vi "st_voltmetr.vi"() -> ()   [LabVIEW 2017]
uses:
  <vilib>/Analysis/4window.llb/windowTd.ctl
  controls/A5000_param.ctl
  subVIs/st_str Global.vi
  <vilib>/measure/maspectr.llb/FFT Spectrum (Mag-Phase) for N Chan.vi
  <vilib>/Utility/file.llb/Read Delimited Spreadsheet (string).vi
  <vilib>/measure/NI_MAPro.lvlib
  <vilib>/Analysis/NI_AALPro.lvlib
panel:
  out "Waveform Spectrogramm":cluster{"f0":dbl, "df":dbl, "magnitude":dbl[]}[](graph)
  in  "window":T1=1 items=["Rectangle"=0, "Hanning"=1, "Hamming"=2, "Blackman-Harris"=3, "Exact Blackman"=4, "Blackman"=5, "Flat Top"=6, "4 Term B-Harris "=7, "7 Term B-Harris"=8, "Low Sidelobe"=9, "Blackman Nuttall"=11, "Triangle"=30, "Bartlett-Hanning"=31, "Bohman"=32, "Parzen"=33, "Welch"=34, "Kaiser"=60, "Dolph-Chebyshev"=61, "Gaussian"=62]
  out "comm?":bool
  out "ItemTag":string
  out "substring before match":string
  out "ItemPath":string
  in  "VChGEN":dbl=0.03 caption="Uскз канал \"GEN\", В" min=0.02 max=1.0 step=0.01 format="%.2f"
  in  "FGen":dbl=10.0 caption="Частота, кГц" min=0.01 max=500.0 step=0.01 format="%_4g"
  in  "GenEnb":bool
  in  "AutoFindFreqChB":bool
  in  "AutoFindFreqChA":bool
  in  "FChB":dbl=10.0 caption="Частота \"B\", кГц" format="%_4g"
  in  "FChA":dbl=10.0 caption="Частота \"A\", кГц" min=0.01 max=500.0 step=0.01 format="%_4g"
  out "VChB":dbl caption="Uскз канал \"B\", В" format="%.3f"
  out "VChA":dbl caption="Uскз канал \"A\", В" format="%.3f"
  in  "RangeChB":T2(ring)=enum."10 В" caption="Диапазон \"B\""
  in  "RangeChA":T3(ring)=enum."10 В" caption="Диапазон \"A\""
  in  "View":T4(ring)
  in  "Protocol":string[][](table)=[["11.02.26 11:54:00", "3.0012e-3", "3.0012e-3", "125,65", "125,65", "1 В", "1 В"], ["", "", "", "", "", "", ""]]
  in  "Checkbox":bool
  out "Waveform Oscillogram":waveform(dbl)[](graph)
  in  "Stop":bool
  in  "Capture":bool=TRUE
  out "overflow":i16
  out "noOfSamples":u32
  in  "Capture":bool
  in  "Tab Control":enum32{"Page 1"}(tab)
  out "OscCon":bool
  in  "Save":bool
  in  "Remove":bool
  in  "Add":bool
  in  "Report":bool
  in  "Delete":bool
  in  "Start Tool":bool
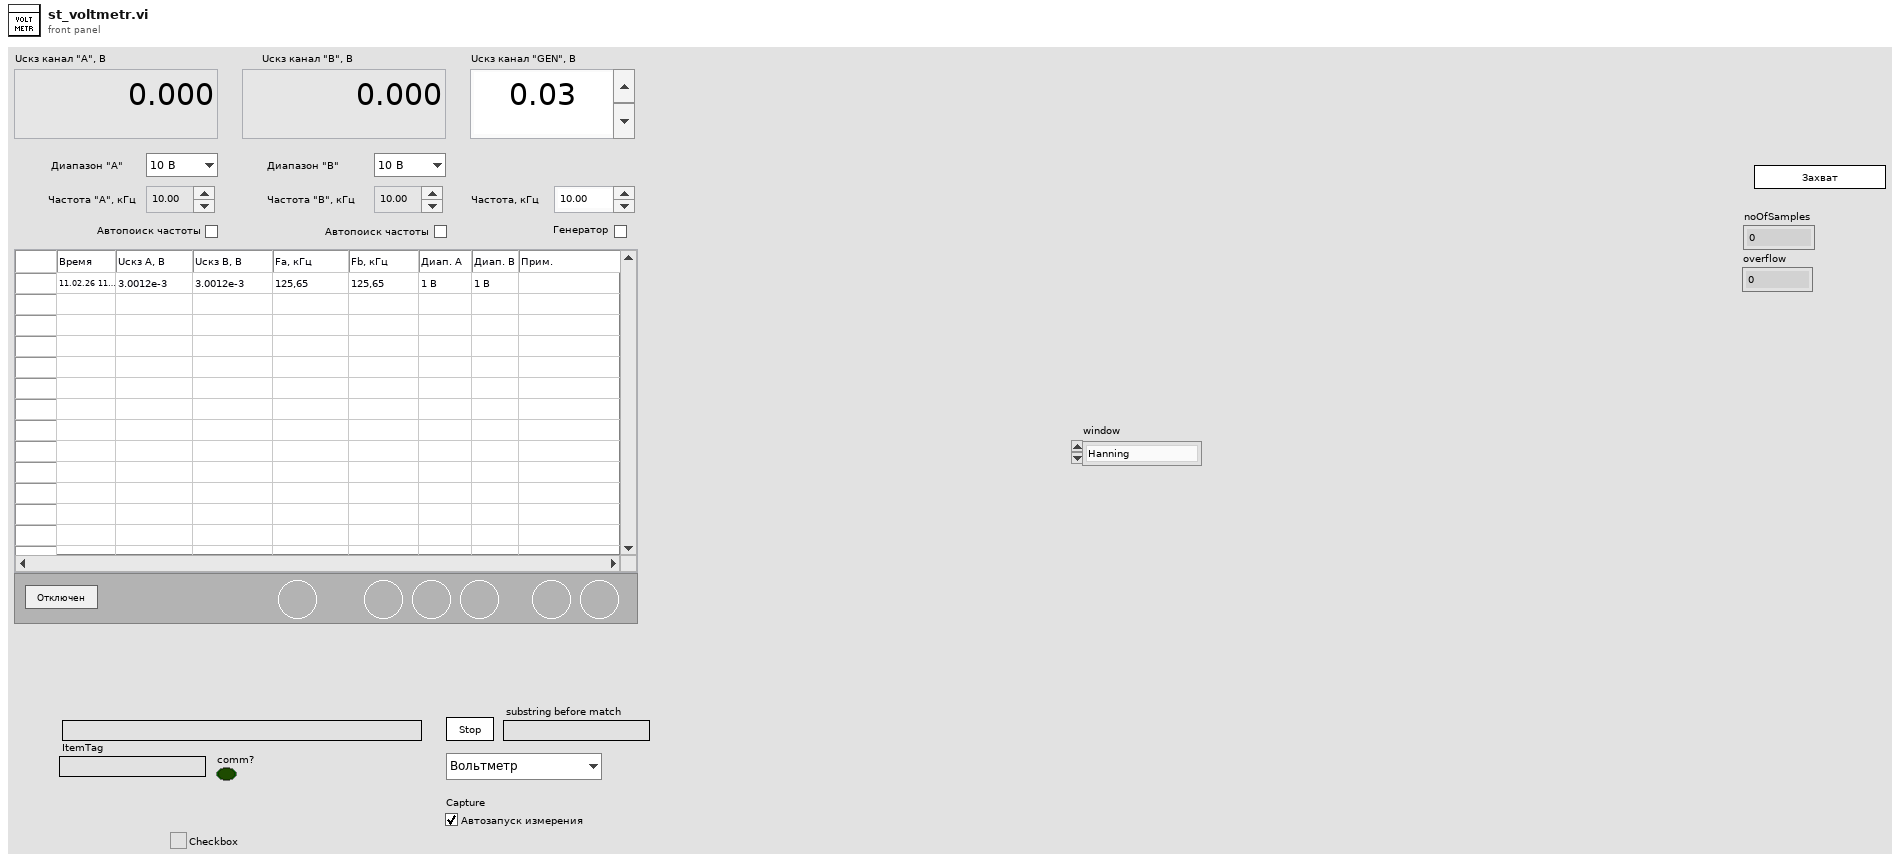
[diagram p1: front panel]
types:
  T1 = typedef "NI_AALPro.lvlib/windowTd.ctl" = u32
  T2 = enum16{"5 мВ", "10 мВ", "25 мВ", "50 мВ", "100 мВ", "250 мВ", "0,5 В", "1 В", "2,5 В", "5 В", "10 В", "Авто", "Выкл."}
  T3 = enum16{"5 мВ", "10 мВ", "25 мВ", "50 мВ", "100 мВ", "250 мВ", "0,5 В", "1,0 В", "2,5 В", "5 В", "10 В", "Авто", "Выкл."}
  T4 = enum16{"Вольтметр", "Осциллограмма", "Спектрограмма"}
  T5 = typedef "A5000_param.ctl" = cluster{"ChannelA":cluster{"Enabled":bool, "Coupling":i16, "Range":u16, "Analogue Offset":sgl}, "ChannelB":cluster{"Enabled":bool, "Coupling":i16, "Range":u16, "Analogue Offset":sgl}, "Trigger":cluster{"Trigger Enabled":bool, "Trigger Source":enum16{"Channel A", "Channel B", "Channel C", "Channel D", "Ext."}, "Trigger Threshold (volts)":dbl, "Trigger Direction":u16, "Trigger Delay (samples)":u32, "Auto Trigger Time (ms)":i16}, "MaxADCvalue":i16, "handle":i16, "Acquisition":cluster{"preTriggerSamples":i32, "postTriggerSamples":i32, "timebase":u32, "Down-Sample Mode":u32, "Down Sample Ratio":u32}, "Device Info":cluster{"Driver Version":string, "USB Version":string, "Hardware":string, "Variant":string, "Batch and Serial":string, "Cal Date":string, "Kernel Version":string, "Digital HW Version":string, "Analogue HW Version":string, "MSO":bool, "Number of channels":i16}, "Properties":cluster{"Sample Frequency":sgl, "Sample Rate":sgl, "Max Samples Available":i32, "Number of Samples":u32, "Total Capture Time (sec) ":sgl, "Max Total Capture Time Available (sec)":sgl}, "Resolution":i32, "EmulateV":bool, "General AWG Settings":cluster{"Peak-to-Peak Voltage (microvolts)":u32, "Offset Voltage (microvolts)":i32, "Wave Type":u32, "Sweep Type":u32, "Shots":u32, "Sweeps":u32, "Trigger Type":u32, "Trigger Source":u32, "Ext. Threshold (ADC count)":i16, "White Noise/PRBS":u32}, "Standard Waveform Settings":cluster{"Start Frequency":dbl, "Stop Frequency":dbl, "Increment":dbl, "Dwell Time (seconds)":dbl}, "Arbitrary Waveform Settings":cluster{"Arbirary waveform file path":path, "Index Mode":u32}, "AutoDiapChA":bool, "AutoDiapChB":bool}
  T6 = cluster{"AutoFindFreqChA":bool, "AutoFindFreqChB":bool, "FChA":dbl, "FChB":dbl}
  T7 = cluster{"dB On (F)":bool, "unwrap phase (F)":bool, "convert to degree (F)":bool}
  T8 = enum8{"Enabled", "Disabled", "Disabled and Grayed Out"}
  T9 = cluster{"Версия:":string, "Наименование ПО:":string, "Год выпуска:":string, "Производитель:":string, "MD5":string, "Наименование ПО полное:":string, "Build":string}
  T10 = typedef "LVRowAndColumnTypeDef.ctl" = cluster{"Row":i32, "Column":i32}
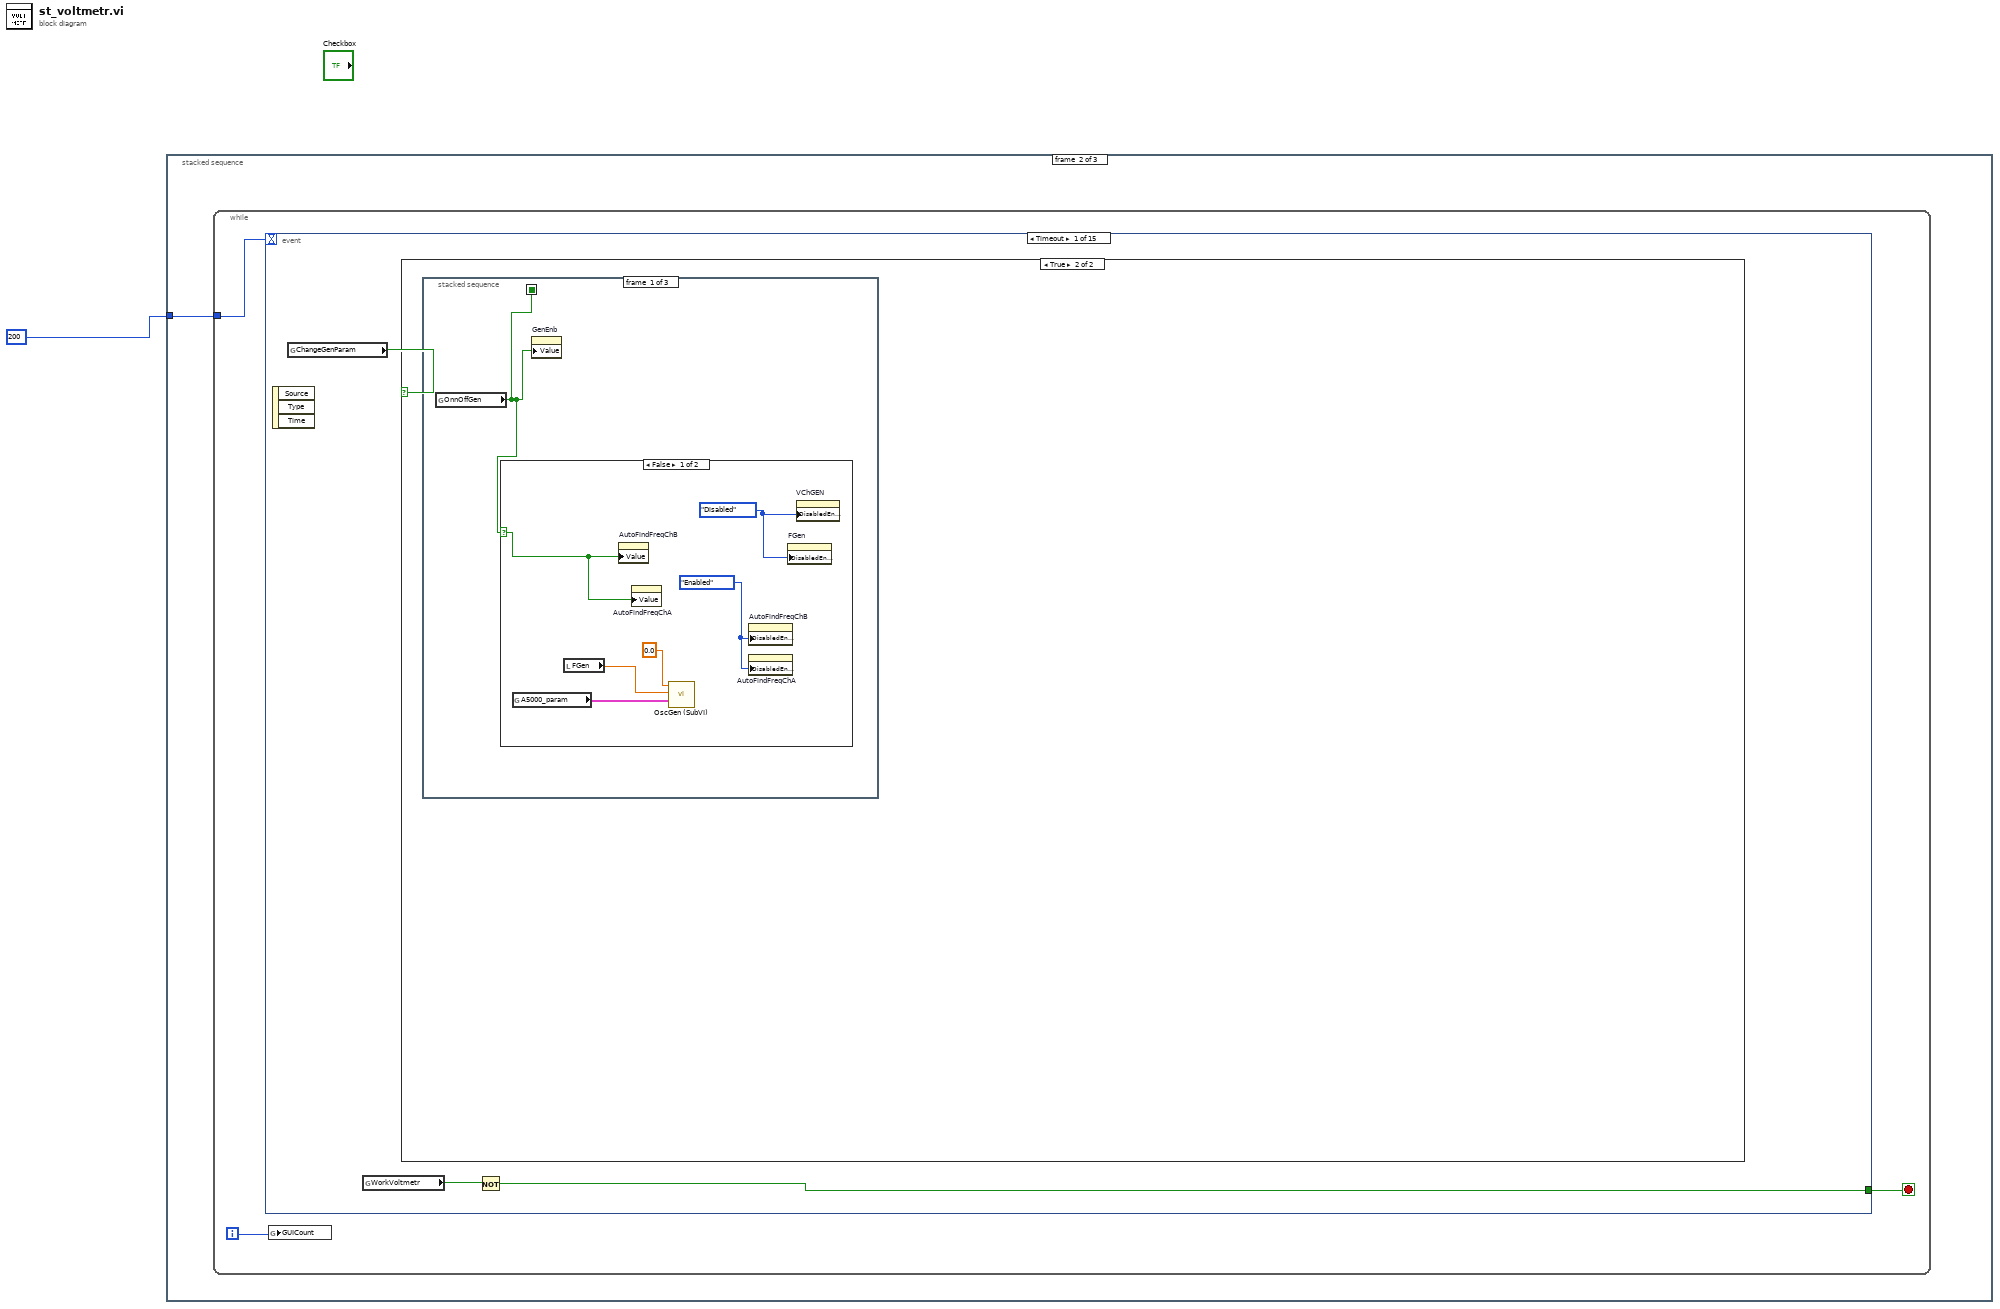
[diagram p0: block diagram]
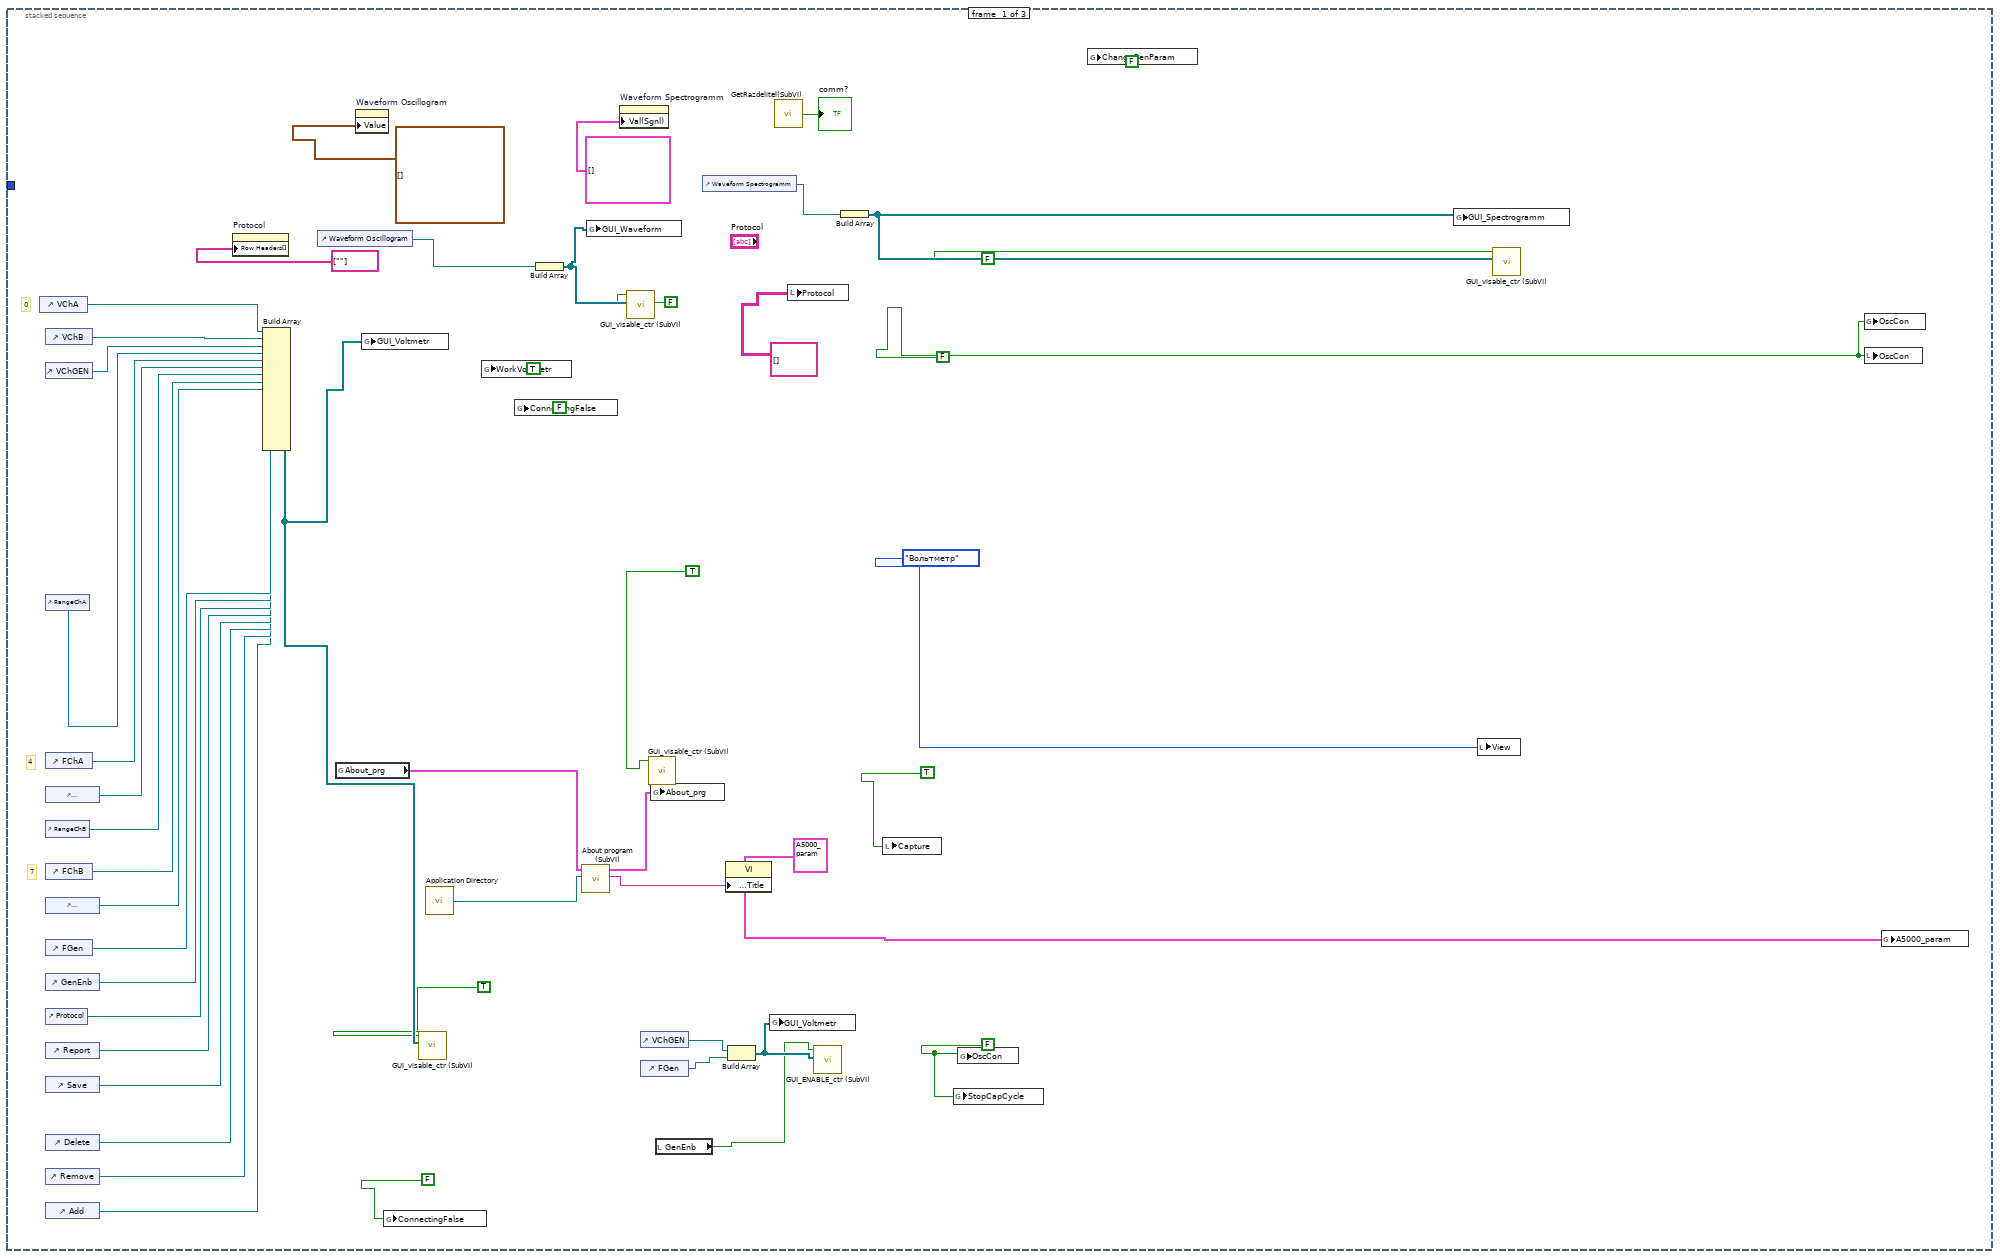
[diagram p2: hidden frame]
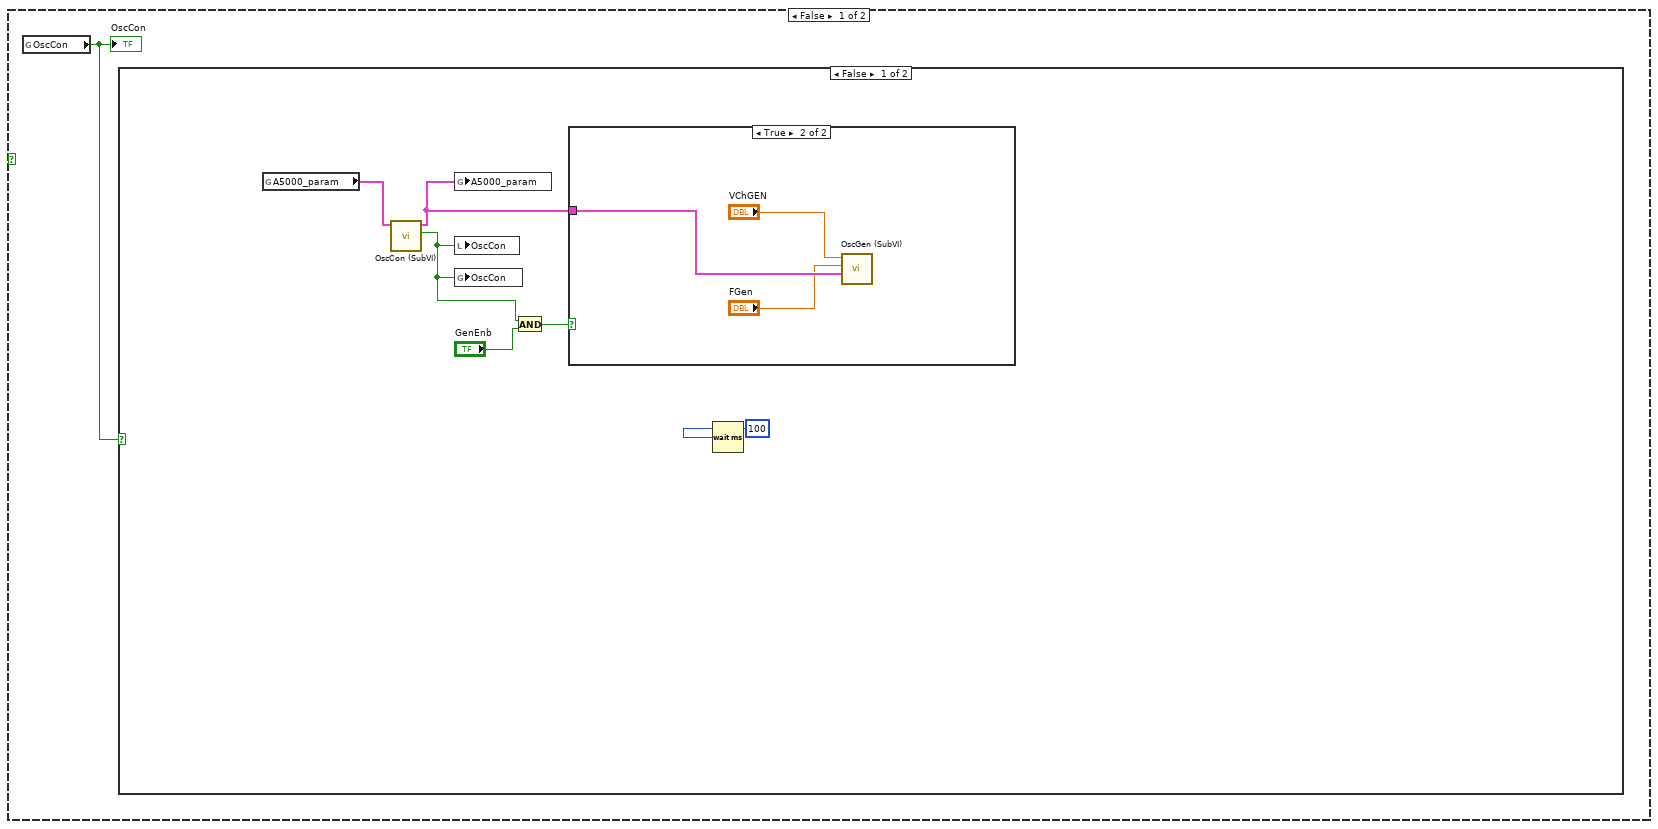
[diagram p3: hidden frame]
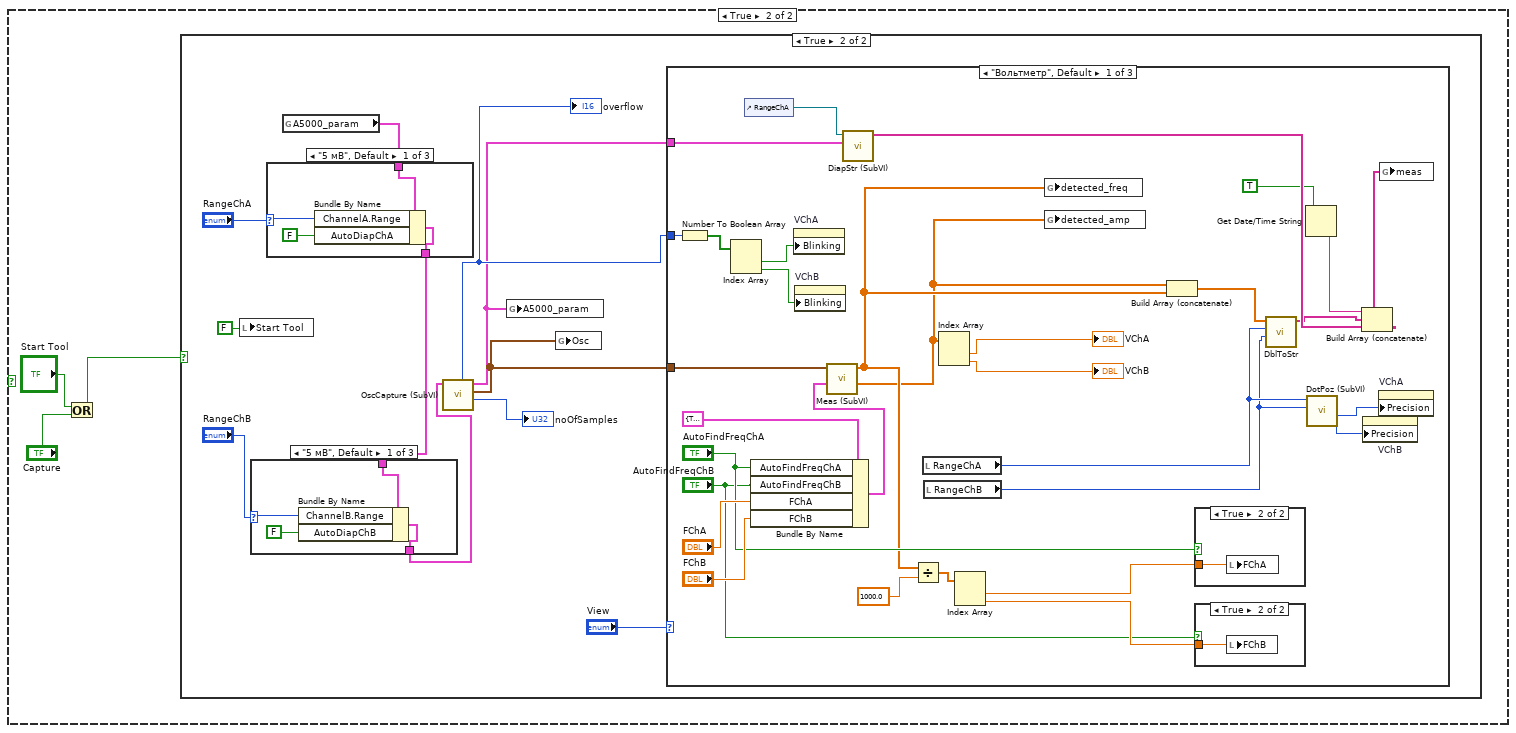
[diagram p5: hidden frame]
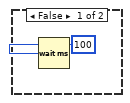
[diagram p6: hidden frame]
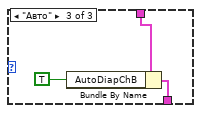
[diagram p8: hidden frame]
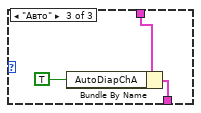
[diagram p10: hidden frame]
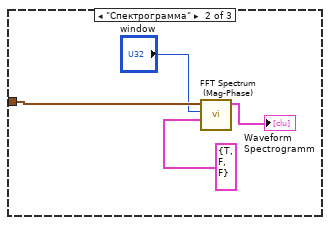
[diagram p13: hidden frame]
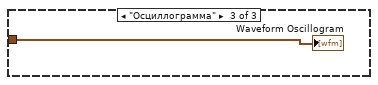
[diagram p14: hidden frame]
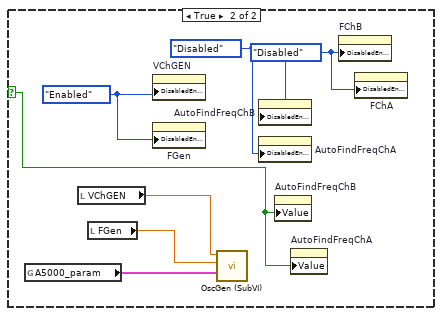
[diagram p15: hidden frame]
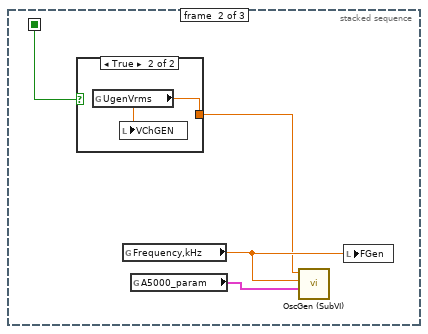
[diagram p16: hidden frame]
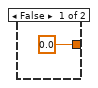
[diagram p17: hidden frame]
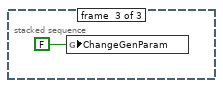
[diagram p18: hidden frame]
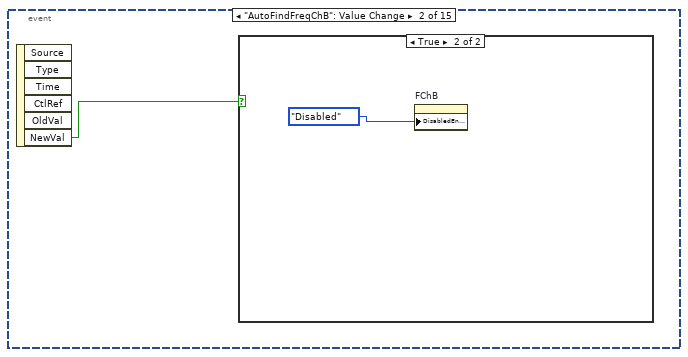
[diagram p19: hidden frame]
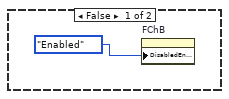
[diagram p20: hidden frame]
diagram:
  n1 = stacked-sequence {
    tunnel: 200 -> [_ w50 _]
    frame #0 {
      w3 = FALSE ("StopCapCycle")
      w49 = FALSE ("OscCon")
      # "0"
      # "7"
      # "4"
      n2 = control-ref of="VChA"() -> (w8:refnum<vi>)
      n3 = control-ref of="VChB"() -> (w47:refnum<vi>)
      n4 = control-ref of="VChGEN"() -> (w46:refnum<vi>)
      n5 = control-ref of="RangeChA"() -> (w45:refnum<vi>)
      n6 = control-ref of="FChA"() -> (w44:refnum<vi>)
      n7 = control-ref of="AutoFindFreqChA"() -> (w43:refnum<vi>)
      n8 = control-ref of="RangeChB"() -> (w42:refnum<vi>)
      n9 = control-ref of="FChB"() -> (w41:refnum<vi>)
      n10 = control-ref of="AutoFindFreqChB"() -> (w40:refnum<vi>)
      n11 = control-ref of="FGen"() -> (w39:refnum<vi>)
      n12 = control-ref of="GenEnb"() -> (w38:refnum<vi>)
      n13 = control-ref of="Protocol"() -> (w29:refnum<vi>)
      n14 = control-ref of="Report"() -> (w25:refnum<vi>)
      n15 = control-ref of="Save"() -> (w24:refnum<vi>)
      n16 = control-ref of="Delete"() -> (w23:refnum<vi>)
      n17 = control-ref of="Remove"() -> (w22:refnum<vi>)
      n18 = control-ref of="Add"() -> (w21:refnum<vi>)
      n19 = property on="Protocol" class="Tbl (strict)"("Row Headers[]"=string[] [""] ("Row Header Strings[]")) -> ()  [unwired: 2 in, 2 out]
      n20 = Build Array(w8, w47, w46, w45, w44, w43, w42, w41, w40, w39, w38, w29, w25, w24, w23, w22, w21) -> (w33:refnum<vi>[])
      n21 = control-ref of="Waveform Oscillogram"() -> (w30:refnum<vi>)
      n22 = global read "st_str Global.vi" "About_prg"() -> (w37:T9)
      n23 = property on="Waveform Oscillogram" class="WFGraph (strict)"("Value"=waveform(dbl)[] [] ("Waveform Oscillogram")) -> ()  [unwired: 2 in, 2 out]
      n24 = global write "st_str Global.vi" "GUI_Voltmetr"(w33) -> ()
      n25 = global write "st_str Global.vi" "ConnectingFalse"(FALSE ("ConnectingFalse")) -> ()
      n26 = call "GUI_visable_ctr (SubVI).vi"("Array"=w33, "Visible"=TRUE) -> ()  [unwired: 9 in, 1 out]
      n27 = call <vilib>:"Application Directory.vi"() -> ("Application Directory"=w35:path)
      n28 = global write "st_str Global.vi" "WorkVoltmetr"(TRUE ("WorkVoltmetr")) -> ()
      n29 = global write "st_str Global.vi" "ConnectingFalse"(FALSE ("ConnectingFalse")) -> ()
      n30 = Build Array(w30) -> (w10:refnum<vi>[])
      n31 = call "About program (SubVI).vi"("Application Directory"=w35, "EC_About_prg in"=w37) -> ("String"=w34:string, "EC_About_prg out"=w36:T9)  [unwired: 8 in]
      n32 = global write "st_str Global.vi" "GUI_Waveform"(w10) -> ()
      n33 = property on="Waveform Spectrogramm" class="WFGraph (strict)"("Val(Sgnl)"=cluster{"f0":dbl, "df":dbl, "magnitude":dbl[]}[] [] ("Value (Signaling)")) -> ()  [unwired: 2 in, 2 out]
      n34 = call "GUI_visable_ctr (SubVI).vi"("Array"=w10, "Visible"=FALSE) -> ()  [unwired: 9 in, 1 out]
      n35 = control-ref of="VChGEN"() -> (w17:refnum<vi>)
      n36 = control-ref of="FGen"() -> (w16:refnum<vi>)
      n37 = call "GUI_visable_ctr (SubVI).vi"("Visible"=TRUE) -> ()  [unwired: 10 in, 1 out]
      n38 = global write "st_str Global.vi" "About_prg"(w36) -> ()
      n39 = local read "GenEnb"() -> (w13:bool)
      n40 = control-ref of="Waveform Spectrogramm"() -> (w27:refnum<vi>)
      n41 = property class="VI"("Front Panel.Title"=w34) -> ()  [unwired: 2 in, 2 out]
      n42 = Build Array(w17, w16) -> (w14:refnum<vi>[])
      n43 = global write "st_str Global.vi" "GUI_Voltmetr"(w14) -> ()
      n44 = call "GetRazdelitel(SubVI).vi"() -> ("comm?"=→"comm?":bool)  [unwired: 1 in]
      n45 = local write "Protocol"(string[][] [] ("Protocol")) -> ()
      n46 = call "GUI_ENABLE_ctr (SubVI).vi"("Array"=w14, "Visible"=w13) -> ()  [unwired: 9 in, 1 out]
      n47 = Build Array(w27) -> (w12:refnum<vi>[])
      n48 = local write "Capture"(TRUE ("Capture")) -> ()
      n49 = global write "st_str Global.vi" "StopCapCycle"(w3) -> ()
      n50 = global write "st_str Global.vi" "OscCon"(w3) -> ()
      n51 = global write "st_str Global.vi" "ChangeGenParam"(FALSE ("ChangeGenParam")) -> ()
      n52 = global write "st_str Global.vi" "GUI_Spectrogramm"(w12) -> ()
      n53 = local write "View"(T4."Вольтметр" ("View")) -> ()
      n54 = call "GUI_visable_ctr (SubVI).vi"("Array"=w12, "Visible"=FALSE) -> ()  [unwired: 9 in, 1 out]
      n55 = global write "st_str Global.vi" "OscCon"(w49) -> ()
      n56 = local write "OscCon"(w49) -> ()
      n57 = global write "st_str Global.vi" "A5000_param"(T5 {"ChannelA"={"Enabled"=TRUE, "Coupling"=1, "Range"=6, "Analogue Offset"=0.0}, "ChannelB"={"Enabled"=TRUE, "Coupling"=1, "Range"=6, "Analogue Offset"=0.0}, "Trigger"={"Trigger Enabled"=FALSE, "Trigger Source"=enum."Channel A", "Trigger Threshold (volts)"=0.0, "Trigger Direction"=2, "Trigger Delay (samples)"=0, "Auto Trigger Time (ms)"=1000}, "MaxADCvalue"=0, "handle"=0, "Acquisition"={"preTriggerSamples"=0, "postTriggerSamples"=12500000, "timebase"=4, "Down-Sample Mode"=2, "Down Sample Ratio"=10}, "Device Info"={"Driver Version"="", "USB Version"="", "Hardware"="", "Variant"="", "Batch and Serial"="", "Cal Date"="", "Kernel Version"="", "Digital HW Version"="", "Analogue HW Version"="", "MSO"=FALSE, "Number of channels"=0}, "Properties"={"Sample Frequency"=0.0, "Sample Rate"=0.0, "Max Samples Available"=0, "Number of Samples"=0, "Total Capture Time (sec) "=0.0, "Max Total Capture Time Available (sec)"=0.0}, "Resolution"=3, "EmulateV"=FALSE, "General AWG Settings"={"Peak-to-Peak Voltage (microvolts)"=2000000, "Offset Voltage (microvolts)"=0, "Wave Type"=0, "Sweep Type"=0, "Shots"=0, "Sweeps"=0, "Trigger Type"=0, "Trigger Source"=0, "Ext. Threshold (ADC count)"=0, "White Noise/PRBS"=0}, "Standard Waveform Settings"={"Start Frequency"=1000.0, "Stop Frequency"=1000.0, "Increment"=0.0, "Dwell Time (seconds)"=0.0}, "Arbitrary Waveform Settings"={"Arbirary waveform file path"=path "", "Index Mode"=0}, "AutoDiapChA"=FALSE, "AutoDiapChB"=FALSE} ("A5000_param")) -> ()
    }
    frame #1 {
      n58 = while {
        tunnel: w50 -> [w52]
        i -> [w51]
        stop <- w53 stop-if-true
        n59 = event shown="[0] Timeout" {
          selector: _ -> [_ _ _ _ _ _ _ _ _ _ _ _ _ _ _]
          dyn-events: _ -> [_ _ _ _ _ _ _ _ _ _ _ _ _ _ _]
          timeout: w52 -> [_ _ _ _ _ _ _ _ _ _ _ _ _ _ _]
          tunnel: [w54 _ _ _ _ TRUE ("Stop") w165 FALSE ("Stop") "Stop" FALSE ("Stop") FALSE ("Stop") _ FALSE ("Stop") FALSE ("Stop") _] -> w53
          event Timeout {
            n60 = event-data() -> ()  [unwired: 1 in, 3 out]
            n61 = global read "st_str Global.vi" "ChangeGenParam"() -> (w56:bool)
            n62 = global read "st_str Global.vi" "WorkVoltmetr"() -> (w55:bool)
            n63 = case shown="True" w56 {
              frame False {
                n64 = global read "st_str Global.vi" "OscCon"() -> (w57:bool)
                "OscCon" <- w57
                n65 = case shown="False" w57 {
                  frame False {
                    n66 = global read "st_str Global.vi" "A5000_param"() -> (w62:T5)
                    n67 = call "OscCon (SubVI).vi"("A5000_param"=w62) -> ("Connect"=w60:bool, "A5000_param_out"=w61:T5)  [unwired: 8 in, 1 out]
                    n68 = global write "st_str Global.vi" "A5000_param"(w61) -> ()
                    n69 = local write "OscCon"(w60) -> ()
                    n70 = global write "st_str Global.vi" "OscCon"(w60) -> ()
                    n71 = And(x=w60, y="GenEnb") -> (x .and. y?=w59:bool)
                    n72 = case shown="True" w59 {
                      tunnel: w61 -> [_ w66]
                      frame False {
                      }
                      frame True {
                        n73 = call "OscGen (SubVI).vi"("A5000_param_out"=w66, "Frequency,kHz"="FGen", "UgenVrms"="VChGEN") -> ()  [unwired: 8 in, 1 out]
                      }
                    }
                    n74 = Wait (ms)(milliseconds to wait=u32 100) -> ()  [unwired: 1 out]
                  }
                  frame True {
                    n75 = Or(x="Start Tool", y="Capture") -> (x .or. y?=w67:bool)
                    n76 = case shown="True" w67 {
                      frame False {
                        n77 = Wait (ms)(milliseconds to wait=u32 100) -> ()  [unwired: 1 out]
                      }
                      frame True {
                        n78 = local write "Start Tool"(FALSE) -> ()
                        n79 = global read "st_str Global.vi" "A5000_param"() -> (w78:T5)
                        n80 = case shown="\"5 мВ\", Default" "RangeChA" {
                          selector: "RangeChA" -> [w93 _ _]
                          tunnel: w78 -> [w92 w94 w97]
                          tunnel: [w91 w94 w95] -> w73
                          frame "5 мВ", Default {
                            n81 = Bundle By Name(cluster=w92, "ChannelA.Range"=w93, "AutoDiapChA"=FALSE) -> (w91:T5)
                          }
                          frame "Выкл." {
                          }
                          frame "Авто" {
                            n82 = Bundle By Name(cluster=w97, "AutoDiapChA"=TRUE) -> (w95:T5)
                          }
                        }
                        n83 = case shown="\"5 мВ\", Default" "RangeChB" {
                          selector: "RangeChB" -> [w85 _ _]
                          tunnel: w73 -> [w84 w86 w89]
                          tunnel: [w83 w86 w87] -> w72
                          frame "5 мВ", Default {
                            n84 = Bundle By Name(cluster=w84, "ChannelB.Range"=w85, "AutoDiapChB"=FALSE ("AutoDiapChA")) -> (w83:T5)
                          }
                          frame "Выкл." {
                          }
                          frame "Авто" {
                            n85 = Bundle By Name(cluster=w89, "AutoDiapChB"=TRUE ("AutoDiapChA")) -> (w87:T5)
                          }
                        }
                        n86 = call "OscCapture (SubVI).vi"("A5000_param in"=w72) -> ("noOfSamples"=→"noOfSamples":u32, "Array"=w79:waveform(dbl)[], "A5000_param out"=w76:T5, "overflow"=w77:i16)  [unwired: 6 in, 1 out]
                        "overflow" <- w77
                        n87 = global write "st_str Global.vi" "A5000_param"(w76) -> ()
                        n88 = global write "st_str Global.vi" "Osc"(w79) -> ()
                        n89 = case shown="\"Вольтметр\", Default" "View" {
                          tunnel: w79 -> [w120 w134 w135]
                          tunnel: w77 -> [w124 _ _]
                          tunnel: w76 -> [w113 _ _]
                          frame "Вольтметр", Default {
                            n90 = Number To Boolean Array(number=w124) -> (Boolean array=w123:bool[])
                            n91 = Index Array(array=w123) -> (element #1=w122:bool, element #2=w121:bool)  [unwired: 2 in]
                            n92 = control-ref of="RangeChA"() -> (w105:refnum<vi>)
                            n93 = Bundle By Name(cluster=T6 {"AutoFindFreqChA"=TRUE, "AutoFindFreqChB"=TRUE, "FChA"=9.999639373509558, "FChB"=38.44515591543487} ("Param"), "AutoFindFreqChA"="AutoFindFreqChA", "AutoFindFreqChB"="AutoFindFreqChB", "FChA"="FChA", "FChB"="FChB") -> (w116:T6)
                            n94 = property on="VChA" class="DigNum (strict)"("Blinking"=w122) -> ()  [unwired: 2 in, 2 out]
                            n95 = property on="VChB" class="DigNum (strict)"("Blinking"=w121) -> ()  [unwired: 2 in, 2 out]
                            n96 = call "Meas (SubVI).vi"("Param"=w116, "Array in"=w120) -> ("RMS, V"=w98:dbl[], "Freq"=w109:dbl[])  [unwired: 7 in, 1 out]
                            n97 = call "DiapStr (SubVI).vi"("A5000_param in"=w113, "reference"=w105) -> ("DiapStr"=w112:string[])  [unwired: 9 in]
                            n98 = Divide(x=w109, y=1000.0) -> (x/y=w125:dbl[])
                            n99 = local read "RangeChA"() -> (w102:T3)
                            n100 = local read "RangeChB"() -> (w101:T2)
                            n101 = Index Array(array=w98) -> (element #1=→"VChA":dbl, element #2=→"VChB":dbl)  [unwired: 2 in]
                            n102 = Index Array(array=w125) -> (element #1=w127:dbl, element #2=w128:dbl)  [unwired: 2 in]
                            n103 = global write "st_str Global.vi" "detected_freq"(w109) -> ()
                            n104 = global write "st_str Global.vi" "detected_amp"(w98) -> ()
                            n105 = Build Array (concatenate)(w98, w109) -> (w108:dbl[])
                            n106 = case shown="True" "AutoFindFreqChA" {
                              tunnel: w127 -> [_ w130]
                              frame False {
                              }
                              frame True {
                                n107 = local write "FChA"(w130) -> ()
                              }
                            }
                            n108 = case shown="True" "AutoFindFreqChB" {
                              tunnel: w128 -> [_ w129]
                              frame False {
                              }
                              frame True {
                                n109 = local write "FChB"(w129) -> ()
                              }
                            }
                            n110 = call "DblToStr.vi"("RangeChB"=w101, "RangeChA"=w102, "DataDbl"=w108) -> ("Out"=w107:string[])  [unwired: 8 in]
                            n111 = Get Date/Time String(want seconds? (F)=TRUE) -> (time string=w111:string)  [unwired: 2 in, 1 out]
                            n112 = call "DotPoz (SubVI).vi"("RangeChB"=w101, "RangeChA"=w102) -> ("BCol"=w99:i32, "ACol"=w100:i32)  [unwired: 6 in, 2 out]
                            n113 = Build Array (concatenate)(w111, w107, w112) -> (w106:string[])
                            n114 = property on="VChB" class="DigNum (strict)"("Precision"=w99) -> ()  [unwired: 2 in, 2 out]
                            n115 = property on="VChA" class="DigNum (strict)"("Precision"=w100) -> ()  [unwired: 2 in, 2 out]
                            n116 = global write "st_str Global.vi" "meas"(w106) -> ()
                          }
                          frame "Спектрограмма" {
                            n117 = call-poly <vilib>:"FFT Spectrum (Mag-Phase).vi"("view"=T7 {"dB On (F)"=TRUE, "unwrap phase (F)"=FALSE, "convert to degree (F)"=FALSE}, "window"="window", "time signals"=w134) -> ("magnitudes"=→"Waveform Spectrogramm":cluster{"f0":dbl, "df":dbl, "magnitude":dbl[]}[])  [unwired: 4 in, 4 out]
                          }
                          frame "Осциллограмма" {
                            "Waveform Oscillogram" <- w135
                          }
                        }
                      }
                    }
                  }
                }
              }
              frame True {
                n118 = stacked-sequence {
                  seq-local: [w136 _ _] -> [_ w151 _]
                  frame #0 {
                    n119 = global read "st_str Global.vi" "OnnOffGen"() -> (w136:bool)
                    n120 = case shown="False" w136 {
                      selector: w136 -> [w137 w143]
                      frame False {
                        w141 = T8."Enabled" ("Disabled")
                        w142 = T8."Disabled" ("Disabled")
                        n121 = global read "st_str Global.vi" "A5000_param"() -> (w139:T5)
                        n122 = local read "FGen"() -> (w140:dbl)
                        n123 = property on="AutoFindFreqChB" class="Bool (strict)"("Value"=w137) -> ()  [unwired: 2 in, 2 out]
                        n124 = property on="AutoFindFreqChA" class="Bool (strict)"("Value"=w137) -> ()  [unwired: 2 in, 2 out]
                        n125 = call "OscGen (SubVI).vi"("A5000_param_out"=w139, "Frequency,kHz"=w140, "UgenVrms"=0.0) -> ()  [unwired: 8 in, 1 out]
                        n126 = property on="AutoFindFreqChB" class="Bool (strict)"("DisabledEnum"=w141) -> ()  [unwired: 2 in, 2 out]
                        n127 = property on="AutoFindFreqChA" class="Bool (strict)"("DisabledEnum"=w141) -> ()  [unwired: 2 in, 2 out]
                        n128 = property on="FGen" class="DigNum (strict)"("DisabledEnum"=w142) -> ()  [unwired: 2 in, 2 out]
                        n129 = property on="VChGEN" class="DigNum (strict)"("DisabledEnum"=w142) -> ()  [unwired: 2 in, 2 out]
                      }
                      frame True {
                        w144 = T8."Disabled" ("Disabled")
                        w145 = T8."Disabled" ("Disabled")
                        w149 = T8."Enabled" ("Disabled")
                        n130 = global read "st_str Global.vi" "A5000_param"() -> (w146:T5)
                        n131 = local read "VChGEN"() -> (w147:dbl)
                        n132 = local read "FGen"() -> (w148:dbl)
                        n133 = property on="VChGEN" class="DigNum (strict)"("DisabledEnum"=w149) -> ()  [unwired: 2 in, 2 out]
                        n134 = property on="FGen" class="DigNum (strict)"("DisabledEnum"=w149) -> ()  [unwired: 2 in, 2 out]
                        n135 = call "OscGen (SubVI).vi"("A5000_param_out"=w146, "Frequency,kHz"=w148, "UgenVrms"=w147) -> ()  [unwired: 8 in, 1 out]
                        n136 = property on="AutoFindFreqChB" class="Bool (strict)"("DisabledEnum"=w145) -> ()  [unwired: 2 in, 2 out]
                        n137 = property on="AutoFindFreqChA" class="Bool (strict)"("DisabledEnum"=w145) -> ()  [unwired: 2 in, 2 out]
                        n138 = property on="AutoFindFreqChB" class="Bool (strict)"("Value"=w143) -> ()  [unwired: 2 in, 2 out]
                        n139 = property on="AutoFindFreqChA" class="Bool (strict)"("Value"=w143) -> ()  [unwired: 2 in, 2 out]
                        n140 = property on="FChB" class="DigNum (strict)"("DisabledEnum"=w144) -> ()  [unwired: 2 in, 2 out]
                        n141 = property on="FChA" class="DigNum (strict)"("DisabledEnum"=w144) -> ()  [unwired: 2 in, 2 out]
                      }
                    }
                    n142 = property on="GenEnb" class="Bool (strict)"("Value"=w136) -> ()  [unwired: 2 in, 2 out]
                  }
                  frame #1 {
                    n143 = case shown="True" w151 {
                      tunnel: [0.0 ("UgenVrms") w155] -> w150
                      frame False {
                      }
                      frame True {
                        n144 = global read "st_str Global.vi" "UgenVrms"() -> (w155:dbl)
                        n145 = local write "VChGEN"(w155) -> ()
                      }
                    }
                    n146 = global read "st_str Global.vi" "Frequency,kHz"() -> (w152:dbl)
                    n147 = global read "st_str Global.vi" "A5000_param"() -> (w153:T5)
                    n148 = call "OscGen (SubVI).vi"("A5000_param_out"=w153, "Frequency,kHz"=w152, "UgenVrms"=w150) -> ()  [unwired: 8 in, 1 out]
                    n149 = local write "FGen"(w152) -> ()
                  }
                  frame #2 {
                    n150 = global write "st_str Global.vi" "ChangeGenParam"(FALSE ("ChangeGenParam")) -> ()
                  }
                }
              }
            }
            n151 = Not(x=w55) -> (.not. x?=w54:bool)
          }
          event "AutoFindFreqChB": Value Change {
            n152 = event-data() -> ("NewVal"=w157:bool)  [unwired: 1 in, 5 out]
            n153 = case shown="True" w157 {
              frame False {
                n154 = property on="FChB" class="DigNum (strict)"("DisabledEnum"=T8."Enabled" ("Disabled")) -> ()  [unwired: 2 in, 2 out]
              }
              frame True {
                n155 = property on="FChB" class="DigNum (strict)"("DisabledEnum"=T8."Disabled" ("Disabled")) -> ()  [unwired: 2 in, 2 out]
              }
            }
          }
          event "AutoFindFreqChA": Value Change {
            n156 = event-data() -> ("NewVal"=w160:bool)  [unwired: 1 in, 5 out]
            n157 = case shown="True" w160 {
              frame False {
                n158 = property on="FChA" class="DigNum (strict)"("DisabledEnum"=T8."Enabled" ("Disabled")) -> ()  [unwired: 2 in, 2 out]
              }
              frame True {
                n159 = property on="FChA" class="DigNum (strict)"("DisabledEnum"=T8."Disabled" ("Disabled")) -> ()  [unwired: 2 in, 2 out]
              }
            }
          }
          event "Save": Value Change {
            n160 = event-data() -> ()  [unwired: 1 in, 6 out]
            n161 = control-ref of="Protocol"() -> (w163:refnum<vi>)
            n162 = call "SaveVolt (SubVI).vi"("Protocol"=w163) -> ()  [unwired: 11 in]
          }
          event "Report": Value Change {
            n163 = event-data() -> ()  [unwired: 1 in, 6 out]
            n164 = call "1poputkapechat (SubVI).vi"() -> ()  [unwired: 12 in]
          }
          event Application Instance Close? {
            n165 = event-data() -> ()  [unwired: 1 in, 5 out]
            n166 = event-data() -> ()  [unwired: 2 in, 1 out]
          }
          event Menu Selection (User) {
            n167 = event-data() -> ("MenuRef"=w168:refnum<k9>, "ItemTag"=w172:string, "ItemPath"=w174:string)  [unwired: 1 in, 4 out]
            "ItemPath" <- w174
            "ItemTag" <- w172
            n168 = case shown="\"Вид:Вольтметр\"" w174 {
              tunnel: [_ _ "Вольтметр" ("search string/char (-)") "Осциллограмма" ("search string/char (-)") "Вольтметр" ("search string/char (-)") _ _ _ _ _ _] -> w170
              tunnel: [_ _ "Спектрограмма" ("search string/char (-)") "Спектрограмма" ("search string/char (-)") "Осциллограмма" ("search string/char (-)") _ _ _ _ _ _] -> w169
              tunnel: w168 -> [_ _ w196 w205 w214 _ _ _ _ _ _]
              tunnel: [FALSE ("Stop") _ _ _ _ _ _ _ _ TRUE ("Stop") _] -> w166
              frame "False", Default {
              }
              frame "Справка:О программе" {
                n169 = call <vilib>:"Application Directory.vi"() -> ("Application Directory"=w189:path)
                n170 = global read "st_str Global.vi" "About_prg"() -> (w190:T9)
                n171 = call "About program (SubVI).vi"("Application Directory"=w189, "EC_About_prg in"=w190) -> ("EC_About_prg out"=w188:T9)  [unwired: 8 in, 1 out]
                n172 = global write "st_str Global.vi" "About_prg"(w188) -> ()
                n173 = call "Dialog_about_program_v (SubVI).vi"("Param"=w188) -> ()  [unwired: 11 in]
              }
              frame "Вид:Осциллограмма" {
                w191 = FALSE ("enabled")
                n174 = global read "st_str Global.vi" "GUI_Voltmetr"() -> (w195:refnum<vi>[])
                n175 = global read "st_str Global.vi" "GUI_Spectrogramm"() -> (w193:refnum<vi>[])
                n176 = global read "st_str Global.vi" "GUI_Waveform"() -> (w194:refnum<vi>[])
                n177 = call "GUI_visable_ctr (SubVI).vi"("Array"=w195, "Visible"=w191) -> ()  [unwired: 9 in, 1 out]
                n178 = call "GUI_visable_ctr (SubVI).vi"("Array"=w193, "Visible"=w191) -> ()  [unwired: 9 in, 1 out]
                n179 = call "GUI_visable_ctr (SubVI).vi"("Array"=w194, "Visible"=TRUE) -> ()  [unwired: 9 in, 1 out]
                n180 = call "DisableEnableControlVolt (SubVI).vi"("enabled"=w191, "Menu in"=w196) -> ()  [unwired: 10 in]
                n181 = local write "View"(T4."Осциллограмма" ("View")) -> ()
              }
              frame "Вид:Вольтметр" {
                w200 = FALSE ("Visible")
                w201 = TRUE ("enabled")
                n182 = global read "st_str Global.vi" "GUI_Waveform"() -> (w203:refnum<vi>[])
                n183 = global read "st_str Global.vi" "GUI_Voltmetr"() -> (w202:refnum<vi>[])
                n184 = global read "st_str Global.vi" "GUI_Spectrogramm"() -> (w204:refnum<vi>[])
                n185 = call "GUI_visable_ctr (SubVI).vi"("Array"=w202, "Visible"=w201) -> ()  [unwired: 9 in, 1 out]
                n186 = call "GUI_visable_ctr (SubVI).vi"("Array"=w203, "Visible"=w200) -> ()  [unwired: 9 in, 1 out]
                n187 = call "GUI_visable_ctr (SubVI).vi"("Array"=w204, "Visible"=w200) -> ()  [unwired: 9 in, 1 out]
                n188 = call "DisableEnableControlVolt (SubVI).vi"("enabled"=w201, "Menu in"=w205) -> ()  [unwired: 10 in]
                n189 = local write "View"(T4."Вольтметр" ("View")) -> ()
              }
              frame "Вид:Спектрограмма" {
                w209 = FALSE ("enabled")
                n190 = global read "st_str Global.vi" "GUI_Voltmetr"() -> (w213:refnum<vi>[])
                n191 = global read "st_str Global.vi" "GUI_Spectrogramm"() -> (w211:refnum<vi>[])
                n192 = global read "st_str Global.vi" "GUI_Waveform"() -> (w212:refnum<vi>[])
                n193 = call "GUI_visable_ctr (SubVI).vi"("Array"=w213, "Visible"=w209) -> ()  [unwired: 9 in, 1 out]
                n194 = call "GUI_visable_ctr (SubVI).vi"("Array"=w211, "Visible"=TRUE) -> ()  [unwired: 9 in, 1 out]
                n195 = call "GUI_visable_ctr (SubVI).vi"("Array"=w212, "Visible"=w209) -> ()  [unwired: 9 in, 1 out]
                n196 = call "DisableEnableControlVolt (SubVI).vi"("enabled"=w209, "Menu in"=w214) -> ()  [unwired: 10 in]
                n197 = local write "View"(T4."Спектрограмма" ("View")) -> ()
              }
              frame "Правка:Очистить протокол" {
                n198 = control-ref of="Protocol"() -> (w218:refnum<vi>)
                n199 = call "DeleteFunction (SubVI).vi"("Protocol"=w218) -> ()  [unwired: 11 in]
              }
              frame "Правка:Добавить измерение в протокол" {
                n200 = control-ref of="Protocol"() -> (w219:refnum<vi>)
                n201 = call "AddFunction (SubVI).vi"("Table in"=w219) -> ()  [unwired: 11 in]
              }
              frame "Правка:Удалить измерение из протокола" {
                n202 = control-ref of="Protocol"() -> (w220:refnum<vi>)
                n203 = call "RemoveFunction (SubVI).vi"("Table in"=w220) -> ()  [unwired: 11 in]
              }
              frame "Файл:Сохранить" {
                n204 = local read "View"() -> (w221:T4)
                n205 = case shown="\"Вольтметр\", Default" w221 {
                  frame "Вольтметр", Default {
                    n206 = control-ref of="Protocol"() -> ()  [unwired: 1 out]
                    n207 = call "SaveVolt (SubVI).vi"() -> ()  [unwired: 12 in]
                  }
                  frame "Осциллограмма" {
                  }
                }
              }
              frame "Файл:Выход" {
              }
              frame "Файл:Открыть" {
                n208 = call "File Dialog"("pattern (all files)"="*.txt") -> ("selected path"=w223:path, "cancelled"=w224:bool)  [unwired: 11 in, 2 out]
                n209 = case shown="False" w224 {
                  tunnel: w223 -> [w226 _]
                  frame False {
                    n210 = stacked-sequence {
                      seq-local: [w228 _] -> [_ w234]
                      tunnel: w226 -> [w228 _]
                      frame #0 {
                        n211 = property on="Protocol" class="Tbl (strict)"("Row Headers[]"=string[] []) -> ()  [unwired: 2 in, 2 out]
                      }
                      frame #1 {
                        n212 = control-ref of="Protocol"() -> (w231:refnum<vi>)
                        n213 = call-poly <vilib>:"Read Delimited Spreadsheet.vi"("file path (dialog if empty)"=w234) -> ("all rows"=w229:string[][])  [unwired: 9 in, 5 out]
                        n214 = Array Size(array=w229) -> (size(s)=w233:i32[])
                        n215 = property on="Protocol" class="Tbl (strict)"("Value"=w229) -> ()  [unwired: 2 in, 2 out]
                        n216 = Index Array(array=w233, index=0) -> (element=w230:i32)
                        n217 = for {
                          tunnel: w229 -> [w235] mode=indexing
                          n218 = for {
                            tunnel: w235 -> [w236] mode=indexing
                            n219 = call "Zamena (SubVI).vi"("input string"=w236) -> ()  [unwired: 10 in, 1 out]
                          }
                        }
                        n220 = for {
                          N: w230 -> [_]
                          tunnel: w231 -> [w239]
                          i -> [w238]
                          n221 = Increment(x=w238) -> (x+1=w237:i32)
                          n222 = call "AddNumRow (SubVI).vi"("element"=w237, "Table in"=w239) -> ()  [unwired: 10 in]
                        }
                      }
                    }
                  }
                  frame True {
                  }
                }
              }
            }
            n223 = Search/Split String(string=w174, search string/char (-)=":") -> (substring before match=w171:string)  [unwired: 1 in, 2 out]
            "substring before match" <- w171
            n224 = case shown="\"Вид\"" w171 {
              tunnel: w168 -> [_ w179 w186]
              tunnel: w172 -> [_ w176 w182]
              tunnel: w170 -> [_ w181 _]
              tunnel: w169 -> [_ w180 _]
              frame "False", Default {
              }
              frame "Вид" {
                w177 = FALSE ("enabled")
                w175 = TRUE ("enabled")
                n225 = Set Menu Item Info(6:w177, 7:w181, 9:w175, 11:w179) -> (3:w178:refnum<k9>)  [unwired: 3 in, 1 out]
                n226 = Set Menu Item Info(6:w177, 7:w180, 9:w175, 11:w178) -> ()  [unwired: 3 in, 2 out]
                n227 = Set Menu Item Info(6:w175, 7:w176, 9:w175, 11:w179) -> ()  [unwired: 3 in, 2 out]
              }
              frame "Параметры" {
                n228 = Get Menu Item Info(7:w182, 11:w186) -> (3:w183:refnum<k9>, 4:w185:bool)  [unwired: 1 in, 5 out]
                n229 = Not(x=w185) -> (.not. x?=w184:bool)
                n230 = Set Menu Item Info(6:w184, 7:w182, 11:w183) -> ()  [unwired: 4 in, 2 out]
                n231 = local write "Capture"(w184) -> ()
              }
            }
            n232 = Or(x=FALSE ("Stop"), y=w166) -> (x .or. y?=w165:bool)
          }
          event "Capture": Value Change {
            n233 = event-data() -> ()  [unwired: 1 in, 6 out]
          }
          event "Stop": Value Change {
            n234 = event-data() -> ()  [unwired: 1 in, 6 out]
          }
          event "VChGEN", "FGen", "GenEnb": Value Change {
            n235 = event-data() -> ()  [unwired: 1 in, 6 out]
            n236 = local read "GenEnb"() -> (w243:bool)
            n237 = global read "st_str Global.vi" "OscCon"() -> (w242:bool)
            n238 = And(x=w242, y=w243) -> (x .and. y?=w244:bool)
            n239 = case shown="True" w244 {
              frame False {
                w249 = T8."Enabled" ("Disabled")
                w250 = T8."Disabled" ("Disabled")
                n240 = global read "st_str Global.vi" "A5000_param"() -> (w247:T5)
                n241 = local read "FGen"() -> (w248:dbl)
                n242 = call "OscGen (SubVI).vi"("A5000_param_out"=w247, "Frequency,kHz"=w248, "UgenVrms"=0.0) -> ()  [unwired: 8 in, 1 out]
                n243 = property on="AutoFindFreqChB" class="Bool (strict)"("DisabledEnum"=w249) -> ()  [unwired: 2 in, 2 out]
                n244 = property on="AutoFindFreqChA" class="Bool (strict)"("DisabledEnum"=w249) -> ()  [unwired: 2 in, 2 out]
                n245 = property on="FGen" class="DigNum (strict)"("DisabledEnum"=w250) -> ()  [unwired: 2 in, 2 out]
                n246 = property on="VChGEN" class="DigNum (strict)"("DisabledEnum"=w250) -> ()  [unwired: 2 in, 2 out]
              }
              frame True {
                w251 = T8."Disabled" ("Disabled")
                w252 = TRUE ("AutoFindFreqChB")
                w253 = T8."Disabled" ("Disabled")
                w257 = T8."Enabled" ("Disabled")
                n247 = global read "st_str Global.vi" "A5000_param"() -> (w254:T5)
                n248 = local read "VChGEN"() -> (w255:dbl)
                n249 = local read "FGen"() -> (w256:dbl)
                n250 = property on="VChGEN" class="DigNum (strict)"("DisabledEnum"=w257) -> ()  [unwired: 2 in, 2 out]
                n251 = property on="FGen" class="DigNum (strict)"("DisabledEnum"=w257) -> ()  [unwired: 2 in, 2 out]
                n252 = call "OscGen (SubVI).vi"("A5000_param_out"=w254, "Frequency,kHz"=w256, "UgenVrms"=w255) -> ()  [unwired: 8 in, 1 out]
                n253 = property on="AutoFindFreqChB" class="Bool (strict)"("DisabledEnum"=w253) -> ()  [unwired: 2 in, 2 out]
                n254 = property on="AutoFindFreqChA" class="Bool (strict)"("DisabledEnum"=w253) -> ()  [unwired: 2 in, 2 out]
                n255 = property on="AutoFindFreqChB" class="Bool (strict)"("Value"=w252) -> ()  [unwired: 2 in, 2 out]
                n256 = property on="AutoFindFreqChA" class="Bool (strict)"("Value"=w252) -> ()  [unwired: 2 in, 2 out]
                n257 = property on="FChB" class="DigNum (strict)"("DisabledEnum"=w251) -> ()  [unwired: 2 in, 2 out]
                n258 = property on="FChA" class="DigNum (strict)"("DisabledEnum"=w251) -> ()  [unwired: 2 in, 2 out]
              }
            }
          }
          event "Add": Value Change {
            n259 = event-data() -> ()  [unwired: 1 in, 6 out]
            n260 = local read "RangeChA"() -> (w260:T3)
            n261 = local read "RangeChB"() -> (w259:T2)
            n262 = local read "comm?"() -> (w258:bool)
            n263 = control-ref of="Protocol"() -> (w261:refnum<vi>)
            n264 = call "AddFunction (SubVI).vi"("comm?"=w258, "RangeChB"=w259, "RangeChA"=w260, "Table in"=w261) -> ()  [unwired: 8 in]
          }
          event "Remove": Value Change {
            n265 = event-data() -> ()  [unwired: 1 in, 6 out]
            n266 = control-ref of="Protocol"() -> (w263:refnum<vi>)
            n267 = call "RemoveFunction (SubVI).vi"("Table in"=w263) -> ()  [unwired: 11 in]
          }
          event "Delete": Value Change {
            n268 = event-data() -> ()  [unwired: 1 in, 6 out]
            n269 = control-ref of="Protocol"() -> (w264:refnum<vi>)
            n270 = call "DeleteFunction (SubVI).vi"("Protocol"=w264) -> ()  [unwired: 11 in]
          }
          event "View": Value Change {
            n271 = event-data() -> ("NewVal"=w271:T4)  [unwired: 1 in, 5 out]
            n272 = case shown="\"Осциллограмма\"" w271 {
              tunnel: [TRUE ("Visable?") FALSE ("Visable?") FALSE ("Visable?")] -> w270
              tunnel: [FALSE ("Visable?") FALSE ("Visable?") TRUE ("Visable?")] -> w268
              frame "Вольтметр", Default {
              }
              frame "Спектрограмма" {
              }
              frame "Осциллограмма" {
              }
            }
            n273 = global read "st_str Global.vi" "GUI_Voltmetr"() -> (w269:refnum<vi>[])
            n274 = global read "st_str Global.vi" "GUI_Waveform"() -> (w267:refnum<vi>[])
            n275 = call "st_str Set Visable on Multiple Controls.vi"("Visable?"=w270, "Controls"=w269) -> ()  [unwired: 10 in]
            n276 = call "st_str Set Visable on Multiple Controls.vi"("Visable?"=w268, "Controls"=w267) -> ()  [unwired: 10 in]
          }
          event "Protocol": Key Down? {
            n277 = event-data() -> ()  [unwired: 1 in, 10 out]
            n278 = property on="Protocol" class="Tbl (strict)"() -> ("Row Headers[]"=w287:string[])  [unwired: 2 in, 2 out]
            n279 = property on="Protocol" class="Tbl (strict)"() -> ("Selection Start"=w290:T10)  [unwired: 2 in, 2 out]
            n280 = Delete From Array(array=w287) -> (array with subset deleted=w286:string[])  [unwired: 2 in, 1 out]
            n281 = Unbundle By Name(w290) -> ("Row"=w285:i32, "Column"=w288:i32)
            n282 = Array Size(array=w286) -> (size(s)=w279:i32)
            n283 = Decrement(x=w279) -> (x-1=w278:i32)
            n284 = Less Or Equal?(x=w288, y=6.0) -> (x <= y?=w284:bool)
            n285 = Less Or Equal?(x=w285, y=w278) -> (x <= y?=w282:bool)
            n286 = Not(x=w284) -> (.not. x?=w283:bool)
            n287 = And(x=w282, y=w283) -> (x .and. y?=w281:bool)
            n288 = Not(x=w281) -> (.not. x?=w280:bool)
            n289 = event-data("Discard?"=w280) -> ()  [unwired: 1 in, 1 out]
          }
        }
        n290 = global write "st_str Global.vi" "GUICount"(w51) -> ()
      }
    }
    frame #2 {
      n291 = global write "st_str Global.vi" "StopCapCycle"(TRUE ("StopCapCycle")) -> ()
      n292 = global write "st_str Global.vi" "StopCapCycle"(FALSE ("StopCapCycle")) -> ()
    }
  }
